vi "OxITC503 _Query_ Read AUTO-PID table.vi"(3 "error in":errorcluster, 5 "VISA session in":refnum<visa-resource-name>) -> (0 "error out":errorcluster, 1 "AUTOPID Table out":T1(array[cluster]), 2 "VISA session ou":refnum<visa-resource-name>)   [LabVIEW 2013]
doc: "Queries ITC503's AUTO-PID table. The AUTO-PID table is a 32x4 matrix of real numbers."
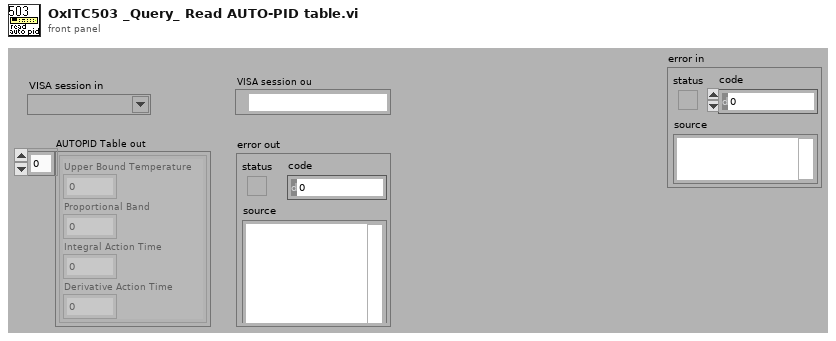
[diagram p1: front panel]
types:
  T1 = cluster{"Upper Bound Temperature":dbl, "Proportional Band":dbl, "Integral Action Time":dbl, "Derivative Action Time":dbl}[]
  T2 = cluster{"Upper Bound Temperature":dbl, "Proportional Band":dbl, "Integral Action Time":dbl, "Derivative Action Time":dbl}
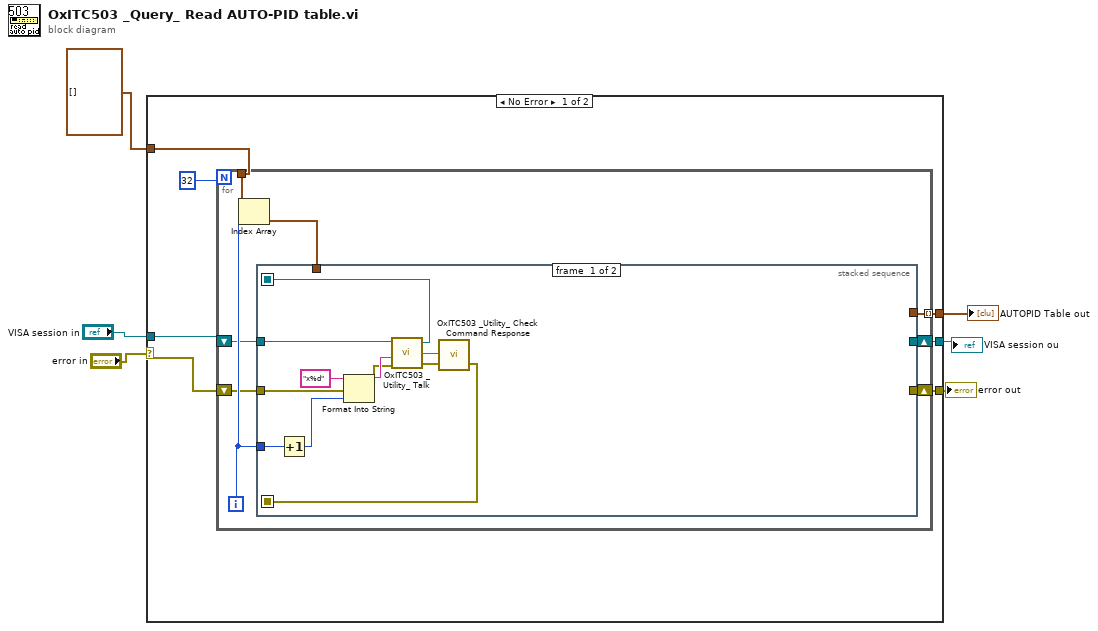
[diagram p0: block diagram]
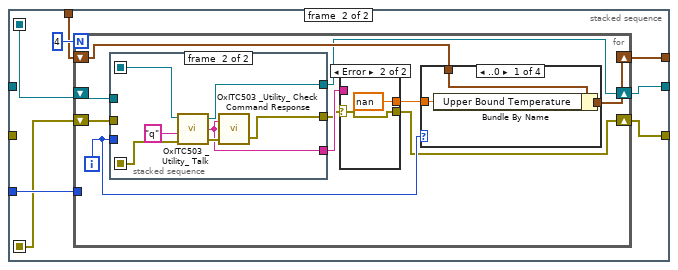
[diagram p2: hidden frame]
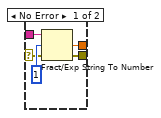
[diagram p3: hidden frame]
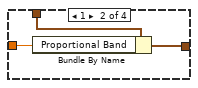
[diagram p4: hidden frame]
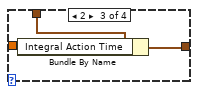
[diagram p5: hidden frame]
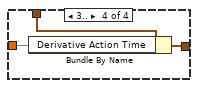
[diagram p6: hidden frame]
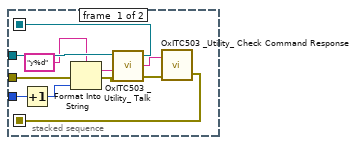
[diagram p7: hidden frame]
diagram:
  n1 = case shown="No Error" "error in" {
    selector: "error in" -> [w8 w88]
    tunnel: [w12 w87] -> w6
    tunnel: [w11 w89] -> w5
    tunnel: [w10 w88] -> w4
    tunnel: "VISA session in" -> [w9 w89]
    tunnel: T1 [] ("AUTOPID Table in") -> [w7 w87]
    frame No Error {
      n2 = for {
        N: 32 -> [_]
        tunnel: w7 -> [w20]
        tunnel: [w19] -> w12 mode=indexing
        shift-right: [w14] -> w10
        shift-left: w8 -> [w17]
        shift-right: [w15] -> w11
        shift-left: w9 -> [w16]
        i -> [w18]
        n3 = Index Array(array=w20, index=w18) -> (element=w21:T2)
        n4 = stacked-sequence {
          seq-local: [w23 _] -> [_ w35]
          seq-local: [w22 _] -> [_ w36]
          tunnel: w18 -> [w32 w39]
          tunnel: w21 -> [_ w37]
          tunnel: [_ w38] -> w19
          tunnel: w17 -> [w26 _]
          tunnel: w16 -> [w24 _]
          tunnel: [_ w34] -> w15
          tunnel: [_ w33] -> w14
          frame #0 {
            n5 = Increment(x=w32) -> (x+1=w25:i32)
            n6 = Format Into String(format string="x%d" ("Format String"), error in=w26, w25) -> (resulting string=w30:string, error out=w27:errorcluster)  [unwired: 1 in]
            n7 = call "OxITC503 _Utility_ Talk.vi"("VISA session"=w24, "Command"=w30, "error in (no error)"=w27) -> ("VISA session"=w23:refnum<visa-resource-name>, "read buffer"=w29:string, "error out (no error)"=w28:errorcluster)  [unwired: 2 in]
            n8 = call "OxITC503 _Utility_ Check Command Response.vi"("error in"=w28, "read buffer"=w29) -> ("error out (no error)"=w22:errorcluster)  [unwired: 1 out]
          }
          frame #1 {
            n9 = for {
              N: 4 -> [_]
              tunnel: w39 -> [_]
              shift-right: [w49] -> w38
              shift-left: w37 -> [w50]
              shift-right: [w42] -> w33
              shift-left: w36 -> [w46]
              shift-right: [w41] -> w34
              shift-left: w35 -> [w45]
              i -> [w48]
              n10 = stacked-sequence {
                seq-local: [w72 _] -> [_ w84]
                seq-local: [w70 _] -> [_ w86]
                tunnel: w48 -> [w79 _]
                tunnel: w46 -> [w74 _]
                tunnel: w45 -> [w73 _]
                tunnel: [_ w82] -> w43
                tunnel: [_ w81] -> w41
                tunnel: [_ w80] -> w44
                frame #0 {
                  n11 = Increment(x=w79) -> (x+1=w75:i32)
                  n12 = Format Into String(format string="y%d" ("Format String"), error in=w74, w75) -> (resulting string=w76:string, error out=w77:errorcluster)  [unwired: 1 in]
                  n13 = call "OxITC503 _Utility_ Talk.vi"("VISA session"=w73, "Command"=w76, "error in (no error)"=w77) -> ("VISA session"=w72:refnum<visa-resource-name>, "read buffer"=w78:string, "error out (no error)"=w71:errorcluster)  [unwired: 2 in]
                  n14 = call "OxITC503 _Utility_ Check Command Response.vi"("error in"=w71, "read buffer"=w78) -> ("error out (no error)"=w70:errorcluster)  [unwired: 1 out]
                }
                frame #1 {
                  n15 = call "OxITC503 _Utility_ Talk.vi"("VISA session"=w84, "Command"="q", "error in (no error)"=w86) -> ("VISA session"=w81:refnum<visa-resource-name>, "read buffer"=w80:string, "error out (no error)"=w83:errorcluster)  [unwired: 2 in]
                  n16 = call "OxITC503 _Utility_ Check Command Response.vi"("error in"=w83, "read buffer"=w80) -> ("error out (no error)"=w82:errorcluster)  [unwired: 1 out]
                }
              }
              n17 = case shown="Error" w43 {
                selector: w43 -> [w51 w55]
                tunnel: [w54 nan] -> w47
                tunnel: w44 -> [w52 _]
                tunnel: [w51 w55] -> w42
                frame No Error {
                  n18 = Fract/Exp String To Number(string=w52, offset=1) -> (number=w54:dbl)  [unwired: 2 in, 1 out]
                }
                frame Error {
                }
              }
              n19 = case shown="..0" w48 {
                tunnel: w50 -> [w59 w61 w64 w67]
                tunnel: w47 -> [w58 w62 w65 w68]
                tunnel: [w57 w60 w63 w66] -> w49
                frame ..0 {
                  n20 = Bundle By Name(cluster=w59, "Upper Bound Temperature"=w58) -> (w57:T2)
                }
                frame 1 {
                  n21 = Bundle By Name(cluster=w61, "Proportional Band"=w62) -> (w60:T2)
                }
                frame 2 {
                  n22 = Bundle By Name(cluster=w64, "Integral Action Time"=w65) -> (w63:T2)
                }
                frame 3.. {
                  n23 = Bundle By Name(cluster=w67, "Derivative Action Time"=w68) -> (w66:T2)
                }
              }
            }
          }
        }
      }
    }
    frame Error {
    }
  }
  "AUTOPID Table out" <- w6
  "VISA session ou" <- w5
  "error out" <- w4
